vi "Day 11.vi"() -> ()   [LabVIEW 2024]
uses:
  <vilib>/Utility/miscctls.llb/LVMapReplaceAction.ctl
panel:
  out "x-y":dbl format="%#_6p"
  out "sum":u64
  in  "Input":string
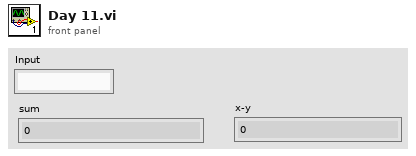
[diagram p1: front panel]
types:
  T1 = typedef "LVMapReplaceAction.ctl" = enum32{"Modify Entry only if found", "Add or Modify Entry", "Delete Entry"}
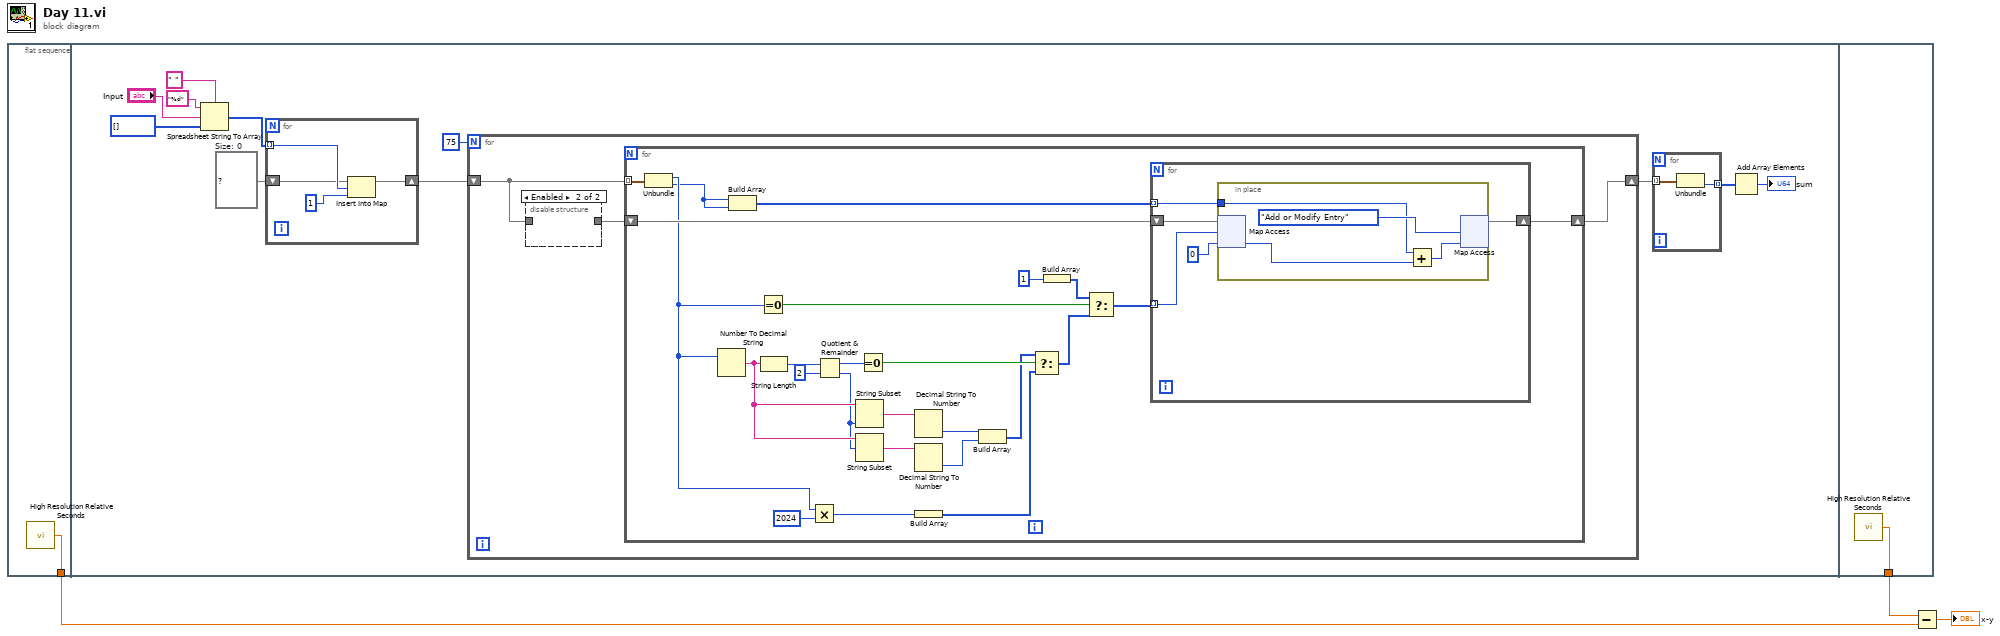
[diagram p0: block diagram]
diagram:
  n1 = flat-sequence {
    tunnel: [w4] -> w2
    tunnel: [w60] -> w3
    frame #0 {
      n2 = call <vilib>:"High Resolution Relative Seconds.vi"() -> ("relative seconds"=w4:dbl)
    }
    frame #1 {
      w13 = map{u64, u64} {}  # Size: 0
      n3 = Spreadsheet String To Array(delimiter (Tab)=" ", format string="%d" ("spreadsheet string"), spreadsheet string="Input", array type (2D Dbl)=u64[] []) -> (array=w14:u64[])
      n4 = for {
        tunnel: w14 -> [w59] mode=indexing
        shift-right: [w57] -> w8
        shift-left: w13 -> [w56]
        n5 = Insert Into Map(map in=w56, key=w59, value=u64 1) -> (map out=w57:map{u64, u64})  [unwired: 2 out]
      }
      n6 = for {
        N: 75 -> [_]
        shift-right: [w16] -> w7
        shift-left: w8 -> [w18]
        n7 = disable-structure shown="Enabled" {
          disable-tunnel: w18 -> [w19 _]
          disable-tunnel: [w19 _] -> w17
          frame Disabled {
          }
          frame Enabled {
          }
        }
        n8 = for {
          tunnel: w18 -> [w43] mode=indexing
          shift-right: [w42] -> w16
          shift-left: w17 -> [w44]
          n9 = Unbundle(w43) -> (w41:u64, w26:u64)
          n10 = Number To Decimal String(number=w41) -> (decimal integer string=w32:string)  [unwired: 1 in]
          n11 = Build Array(w26, w26) -> (w20:u64[])
          n12 = Equal To 0?(x=w41) -> (x = 0?=w40:bool)
          n13 = String Length(string=w32) -> (length=w38:i32)
          n14 = Multiply(x=w41, y=u64 2024) -> (x*y=w23:u64)
          n15 = Quotient & Remainder(x=w38, y=2) -> (x-y*floor(x/y)=w39:i32, floor(x/y)=w31:i32)
          n16 = String Subset(string=w32, length (rest)=w31) -> (substring=w30:string)  [unwired: 1 in]
          n17 = String Subset(string=w32, offset (0)=w31) -> (substring=w29:string)  [unwired: 1 in]
          n18 = Equal To 0?(x=w39) -> (x = 0?=w34:bool)
          n19 = Decimal String To Number(string=w30) -> (number=w28:i32)  [unwired: 2 in, 1 out]
          n20 = Decimal String To Number(string=w29) -> (number=w27:i32)  [unwired: 2 in, 1 out]
          n21 = Build Array(w23) -> (w22:u64[])
          n22 = Build Array(w28, w27) -> (w24:i32[])
          n23 = Select(t=w24, s=w34, f=w22) -> (s? t:f=w33:u64[])
          n24 = Build Array(u64 1) -> (w25:u64[])
          n25 = Select(t=w25, s=w40, f=w33) -> (s? t:f=w21:u64[])
          n26 = for {
            shift-right: [w48] -> w42
            shift-left: w44 -> [w49]
            tunnel: w21 -> [w46] mode=indexing
            tunnel: w20 -> [w45] mode=indexing
            n27 = in-place {
              in-place-border: w45 -> [w50]
              n28 = in-place-map #1(w49, w46, u64 0) -> (w52:u64)  [unwired: 1 out]
              n29 = Add(x=w50, y=w52) -> (x+y=w51:u64)
              n30 = in-place-map #1(w51, LVMapReplaceAction."Add or Modify Entry" ("action")) -> (w48:map{u64, u64})  [unwired: 2 out]
            }
          }
        }
      }
      n31 = for {
        tunnel: w7 -> [w55] mode=indexing
        tunnel: [w54] -> w6 mode=indexing
        n32 = Unbundle(w55) -> (w54:u64)  [unwired: 1 out]
      }
      n33 = Add Array Elements(numeric array=w6) -> (sum=→"sum":u64)
    }
    frame #2 {
      n34 = call <vilib>:"High Resolution Relative Seconds.vi"() -> ("relative seconds"=w60:dbl)
    }
  }
  n35 = Subtract(x=w3, y=w2) -> (x-y=→"x-y":dbl)
